vi "Autonomous Independent.vi"   [LabVIEW 2013]
doc: "This VI is called when autonomous begins, and will automatically be terminated when autonomous ends. You can carry out timed or sensor driven robot movement independently without needing to return to the caller."
uses:
  <vilib>/Rock Robotics/WPI/Relay/WPI_RelayValue.ctl
  <vilib>/Rock Robotics/WPI/Solenoid/WPI_SolenoidValue.ctl
  Robot Global Data.vi
  <vilib>/Rock Robotics/WPI/Solenoid/WPI_SolenoidSetEnum.vi
  <vilib>/Rock Robotics/WPI/RobotDrive/WPI_RobotDriveGetSetRefNum.vi
  <vilib>/Rock Robotics/WPI/Joystick/WPI_JoystickGetSetRefNum.vi
panel:
  # "Be sure to right-click and choose Data Operations>>Make Current Value default if you want to save the array values with the VI"
types:
  T1 = typedef "WPI_JoystickDevRef.ctl" = cluster{"Device":T2}
  T2 = typedef "WPI_JoystickDeviceEnum.ctl" = enum16{"USB 1", "USB 2", "USB 3", "USB 4", "Kinect 1", "Kinect 2"}
  T3 = cluster{"axis 1 (x)":dbl, "axis 2 (y)":dbl, "axis 3 (throttle)":dbl, "axis 4":dbl, "axis 5":dbl, "axis 6":dbl}
  T4 = typedef "WPI_RelayValue.ctl" = enum16{"Off", "On", "Forward", "Reverse"}
  T5 = typedef "WPI_RobotDriveDevRef.ctl" = cluster{"DevStatus":errorcluster, "Motors[]":T6[], "Square Inputs":bool, "Max Output":dbl, "Isochronous":bool}
  T6 = typedef "WPI_MotorControlDeviceRef.ctl" = cluster{"DeviceStatus":errorcluster, "Type":enum16{"PWM", "CAN"}, "PWM":cluster{"Digital Module":T7, "PWM Channel":T8, "DeadBand":T9}, "CAN":cluster{"Device Number":u8, "Control Mode":T10, "Semaphore":T11, "Max Vout":dbl}, "Invert":bool, "TransformRef":T12, "InvTransformRef":T12}
  T7 = typedef "FPGA_TypedefDigitalModule.ctl" = enum16{"Digital Module 1", "Digital Module 2"}
  T8 = typedef "FPGA_DIOPWMChannel.ctl" = enum8{"PWM 1", "PWM 2", "PWM 3", "PWM 4", "PWM 5", "PWM 6", "PWM 7", "PWM 8", "PWM 9", "PWM 10", "Invalid"}
  T9 = typedef "WPI_PWMDeadband.ctl" = cluster{"Name":string, "maxPositivePwm":i32, "minPositivePwm":i32, "centerPwm":i32, "maxNegativePwm":i32, "minNegativePwm":i32, "angularRange":u16}
  T10 = typedef "WPI_CANJaguar_ControlMode.ctl" = enum8{"Percent VBus", "Current", "Speed", "Position", "Voltage"}
  T11 = typedef "Semaphore RefNum" = refnum<k1>
  T12 = typedef "WPI_PWMTransform_ConPane.ctl" = refnum<vi>
  T13 = typedef "WPI_RelayDevRef.ctl" = cluster{"DevStatus":errorcluster, "Relay Channel":T14, "Digital Module":T7, "Relay Direction":T15}
  T14 = typedef "FPGA_DIORelayChannel.ctl" = enum8{"Relay 1", "Relay 2", "Relay 3", "Relay 4", "Relay 5", "Relay 6", "Relay 7", "Relay 8", "Invalid"}
  T15 = typedef "WPI_RelayDirection.ctl" = enum16{"Both directions", "Forward only", "Reverse only"}
  T16 = typedef "WPI_SolenoidValue.ctl" = enum16{"Off", "On", "Forward", "Reverse"}
  T17 = typedef "WPI_SolenoidDevRef.ctl" = cluster{"DevStatus":errorcluster, "Solenoid Module":T18, "Forward Solenoid Channel":T19, "Reverse Solenoid Channel":T19}
  T18 = typedef "FPGA_TypedefSolenoidModule.ctl" = enum16{"Solenoid Module 1", "Solenoid Module 2"}
  T19 = typedef "WPI_SolenoidChannel.ctl" = enum8{"Solenoid 1", "Solenoid 2", "Solenoid 3", "Solenoid 4", "Solenoid 5", "Solenoid 6", "Solenoid 7", "Solenoid 8", "Invalid"}
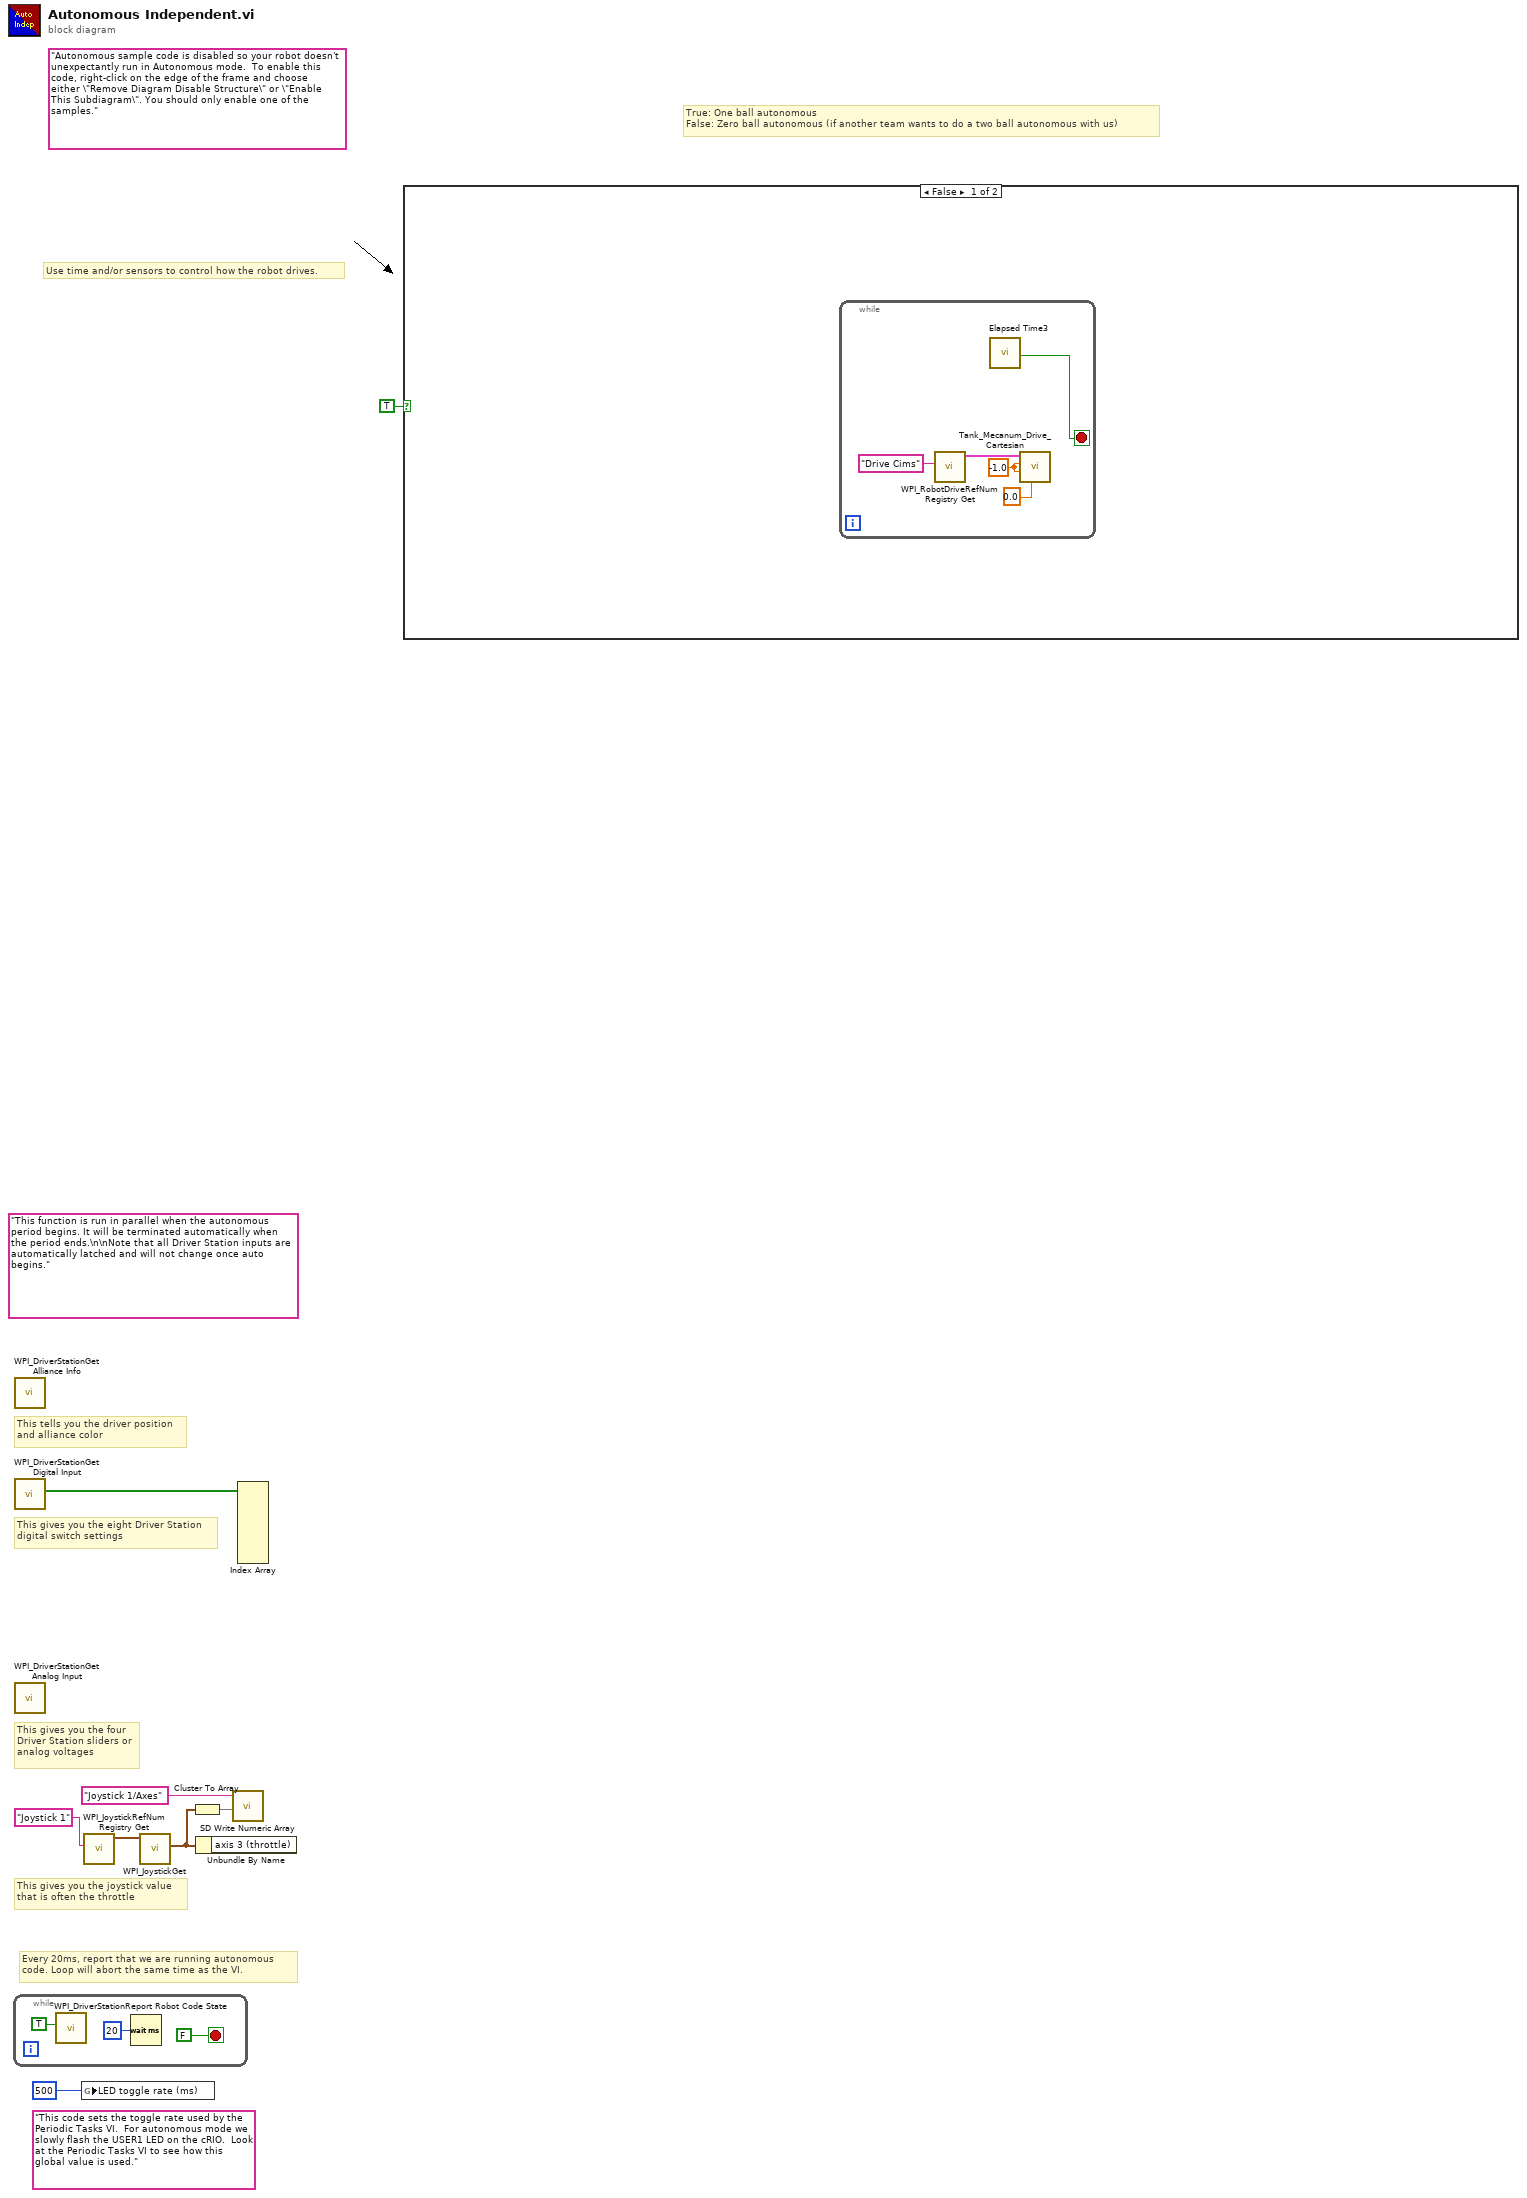
[diagram p0: block diagram]
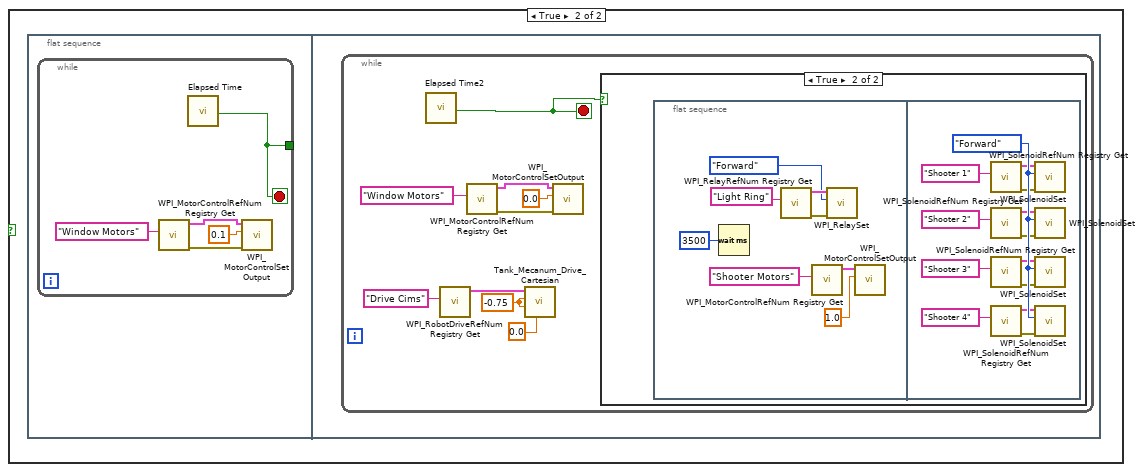
[diagram p2: hidden frame]
diagram:
  (unwired) "This code sets the toggle rate used by the Periodic Tasks VI.  For autonomous mode we slowly flash the USER1 LED on the cRIO.  Look at the Periodic Tasks VI to see how this global value is used."
  (unwired) "Autonomous sample code is disabled so your robot doesn't unexpectantly run in Autonomous mode.  To enable this code, right-click on the edge of the frame and choose either \"Remove Diagram Disable Structure\" or \"Enable This Subdiagram\". You should only enable one of the samples."
  (unwired) "This function is run in parallel when the autonomous period begins. It will be terminated automatically when the period ends.\n\nNote that all Driver Station inputs are automatically latched and will not change once auto begins."
  # "True: One ball autonomous\nFalse: Zero ball autonomous (if another team wants to do a two ball autonomous with us)"
  # "Every 20ms, report that we are running autonomous\ncode. Loop will abort the same time as the VI."
  # "This gives you the joystick value\nthat is often the throttle"
  # "Use time and/or sensors to control how the robot drives."
  # "This tells you the driver position\nand alliance color"
  # "This gives you the eight Driver Station\ndigital switch settings"
  # "This gives you the four\nDriver Station sliders or\nanalog voltages"
  n1 = while {
    stop <- FALSE stop-if-true
    n2 = call <vilib>:"WPI_DriverStationReport Robot Code State.vi"("Autonomous"=TRUE) -> ()  [unwired: 10 in, 1 out]
    n3 = Wait (ms)(milliseconds to wait=u32 20) -> ()  [unwired: 1 out]
  }
  n4 = call <vilib>:"WPI_DriverStationGet Alliance Info.vi"() -> ()  [unwired: 12 out]
  n5 = call <vilib>:"WPI_DriverStationGet Digital Input.vi"() -> ("Driver Station Digital Input (1-8)"=w8:bool[])  [unwired: 11 out]
  n6 = call <vilib>:"WPI_DriverStationGet Analog Input.vi"() -> ()  [unwired: 12 out]
  n7 = global write "Robot Global Data.vi" "LED toggle rate (ms)"(u32 500 ("LED ms toggle rate")) -> ()
  n8 = call <vilib>:"WPI_JoystickRefNum Registry Get.vi"("refnum name"="Joystick 1") -> ("JoystickDevRef"=w6:T1)  [unwired: 1 in, 9 out]
  n9 = call <vilib>:"WPI_JoystickGet.vi"("JoystickDevRef"=w6) -> ("Axes"=w3:T3)  [unwired: 1 in, 5 out]
  n10 = Cluster To Array(cluster=w3) -> (array=w4:dbl[])
  n11 = Unbundle By Name(w3) -> ()  [unwired: 1 out]
  n12 = call <vilib>:"SD Write Numeric Array.vi"("Numeric Array"=w4, "Name"="Joystick 1/Axes") -> ()  [unwired: 8 in, 2 out]
  n13 = Index Array(array=w8) -> ()  [unwired: 8 in, 8 out]
  n14 = case shown="False" TRUE {
    frame False {
      n15 = while {
        stop <- w16 stop-if-true
        w12 = -1.0 ("Y")
        n16 = call <vilib>:"WPI_RobotDriveRefNum Registry Get.vi"("refnum name"="Drive Cims") -> ("RobotDriveDevRef"=w14:T5)  [unwired: 9 in, 1 out]
        n17 = call "Elapsed Time3"() -> ("Time has Elapsed"=w16:bool)  [unwired: 12 in, 7 out]
        n18 = call "Tank_Mecanum_Drive_Cartesian.vi"("Left X"=0.0 ("X"), "Left Y"=w12, "Right Y"=w12, "RobotDriveDevRef"=w14) -> ()  [unwired: 5 in, 3 out]
      }
    }
    frame True {
      n19 = flat-sequence {
        frame #0 {
          n20 = while {
            tunnel: [w17] -> _
            stop <- w17 stop-if-true
            n21 = call <vilib>:"WPI_MotorControlRefNum Registry Get.vi"("refnum name"="Window Motors") -> ("error out"=w19:errorcluster, "MotorControlDevRef"=w20:T6)  [unwired: 9 in]
            n22 = call "Elapsed Time"() -> ("Time has Elapsed"=w17:bool)  [unwired: 12 in, 7 out]
            n23 = call <vilib>:"WPI_MotorControlSetOutput.vi"("error in (no error)"=w19, "Output"=0.1, "MotorControlDevRef"=w20) -> ()  [unwired: 6 in, 3 out]
          }
        }
        frame #1 {
          n24 = while {
            stop <- w30 stop-if-true
            w26 = -0.75 ("Y")
            n25 = call "Elapsed Time2"() -> ("Time has Elapsed"=w30:bool)  [unwired: 12 in, 7 out]
            n26 = call <vilib>:"WPI_RobotDriveRefNum Registry Get.vi"("refnum name"="Drive Cims") -> ("RobotDriveDevRef"=w28:T5)  [unwired: 9 in, 1 out]
            n27 = call <vilib>:"WPI_MotorControlRefNum Registry Get.vi"("refnum name"="Window Motors") -> ("error out"=w24:errorcluster, "MotorControlDevRef"=w23:T6)  [unwired: 9 in]
            n28 = call "Tank_Mecanum_Drive_Cartesian.vi"("Left X"=0.0 ("X"), "Left Y"=w26, "Right Y"=w26, "RobotDriveDevRef"=w28) -> ()  [unwired: 5 in, 3 out]
            n29 = call <vilib>:"WPI_MotorControlSetOutput.vi"("error in (no error)"=w24, "Output"=0.0, "MotorControlDevRef"=w23) -> ()  [unwired: 6 in, 3 out]
            n30 = case shown="True" w30 {
              frame False {
              }
              frame True {
                n31 = flat-sequence {
                  frame #0 {
                    n32 = Wait (ms)(milliseconds to wait=u32 3500) -> ()  [unwired: 1 out]
                    n33 = call <vilib>:"WPI_RelayRefNum Registry Get.vi"("refnum name"="Light Ring") -> ("error out"=w35:errorcluster, "RelayDevRef"=w34:T13)  [unwired: 9 in]
                    n34 = call <vilib>:"WPI_MotorControlRefNum Registry Get.vi"("refnum name"="Shooter Motors") -> ("MotorControlDevRef"=w36:T6)  [unwired: 9 in, 1 out]
                    n35 = call <vilib>:"WPI_RelaySet.vi"("error in (no error)"=w35, "RelayValue"=WPI_RelayValue."Forward", "RelayDevRef"=w34) -> ()  [unwired: 7 in, 2 out]
                    n36 = call <vilib>:"WPI_MotorControlSetOutput.vi"("Output"=1.0, "MotorControlDevRef"=w36) -> ()  [unwired: 7 in, 3 out]
                  }
                  frame #1 {
                    w51 = WPI_SolenoidValue."Forward" ("Value")
                    n37 = call <vilib>:"WPI_SolenoidRefNum Registry Get.vi"("refnum name"="Shooter 1") -> ("error out"=w42:errorcluster, "SolenoidDevRef"=w43:T17)  [unwired: 9 in]
                    n38 = call <vilib>:"WPI_SolenoidRefNum Registry Get.vi"("refnum name"="Shooter 2") -> ("error out"=w39:errorcluster, "SolenoidDevRef"=w40:T17)  [unwired: 9 in]
                    n39 = call <vilib>:"WPI_SolenoidRefNum Registry Get.vi"("refnum name"="Shooter 3") -> ("error out"=w45:errorcluster, "SolenoidDevRef"=w49:T17)  [unwired: 9 in]
                    n40 = call <vilib>:"WPI_SolenoidRefNum Registry Get.vi"("refnum name"="Shooter 4") -> ("error out"=w46:errorcluster, "SolenoidDevRef"=w50:T17)  [unwired: 9 in]
                    n41 = call-poly <vilib>:"WPI_SolenoidSet.vi"("error in (no error)"=w42, "Value"=w51, "SolenoidDevRef"=w43) -> ()  [unwired: 7 in, 2 out]
                    n42 = call-poly <vilib>:"WPI_SolenoidSet.vi"("error in (no error)"=w39, "Value"=w51, "SolenoidDevRef"=w40) -> ()  [unwired: 7 in, 2 out]
                    n43 = call-poly <vilib>:"WPI_SolenoidSet.vi"("error in (no error)"=w45, "Value"=w51, "SolenoidDevRef"=w49) -> ()  [unwired: 7 in, 2 out]
                    n44 = call-poly <vilib>:"WPI_SolenoidSet.vi"("error in (no error)"=w46, "Value"=w51, "SolenoidDevRef"=w50) -> ()  [unwired: 7 in, 2 out]
                  }
                }
              }
            }
          }
        }
      }
    }
  }
